vi "Test-Elevator-Commands.vi"() -> ()   [LabVIEW 2014, in "Comp Elevator.lvlib"]
uses:
  Comp Elevator.lvlib
  Robot/Elevator/Elevator Command/EL-Go to Height/EL-Go To Height Class/Parameters.ctl
  Robot/Elevator/Elevator Class/Elevator State.ctl
  Robot/Elevator/Elevator State Receiver Class/Elevator State Receiver.lvclass
  <vilib>/Rock Robotics/WPI/DriverStation/WPI_DriverStationRobotMode2.ctl
  Robot/Elevator/Elevator State Receiver Messages/Update Elevator State Msg/Update Elevator State Msg.lvclass
  Robot/Elevator/Elevator Messages/Request Current State Msg/Request Current State Msg.lvclass
  Robot/Elevator/Elevator Command/EL-Go to Height/EL-Go To Height Class/EL-Go To Height.lvclass
  Robot Actor Framework/System Actor/System Actor Messages/Start Command Msg/Start Command Msg.lvclass/Start Command Msg.ctl
  <vilib>/ActorFramework/Message Enqueuer/Message Enqueuer.lvclass/Message Enqueuer.ctl
  Robot/Elevator/Elevator Messages/Set Rate (Percent) Msg/Set Rate (Percent) Msg.lvclass/Set Rate (Percent) Msg.ctl
  <vilib>/ActorFramework/Message Enqueuer/Enqueue.vi
  Dev Robot/Robot Global Data.vi
  <vilib>/ActorFramework/Message Priority Queue/Priority Enqueue.vi
  Robot Actor Framework/System Actor/System Actor Messages/Update Tuning from File Msg/Update Tuning from File Msg.lvclass
  Robot Actor Framework/System Actor/System Actor Messages/Start Command Msg/Start Command Msg.lvclass
  Robot/Elevator/Elevator Messages/Set Rate (Percent) Msg/Set Rate (Percent) Msg.lvclass
  Robot Actor Framework/System Actor/System Actor Messages/Stop Command Msg/Stop Command Msg.lvclass
  <vilib>/ActorFramework/Stop Msg/Stop Msg.lvclass
  Robot Actor Framework/Command Actor/Command Actor Class/Command Actor.lvclass
  Robot Actor Framework/Utilities/Utilities.lvlib
  <vilib>/ActorFramework/Actor/Actor.lvclass
  Robot/Elevator/Elevator Class/Elevator.lvclass
panel:
  out "Delivery Notifier Error":errorcluster
  in  "Stop Command":bool=TRUE
  in  "Manual Elevate":enum32{"Up", "Hold", "Down"}(radio)=enum."Hold"
  out "error out":errorcluster
  out "Elevator State":T1 {"Current Elevation" scale=0.0..100.0; "Current Travel Rate" scale=-1.0..1.0}
  out "Start Command error out":errorcluster
  out "Command Running":bool
  in  "Fire Commamd":bool
  in  "Command Parameters":enum32{"No Command", "Go To Height", "Page 2"}(tab)
  in  "EL-GTH-Parameters":T2={"Target Height"=0.0, "Elevator State Loop (ms)"=20, "Up Rate (Percentage)"=1.0, "Down Rate (Percentage)"=-1.0}
  in  "Command":T3(radio)
  in  "Test Loop":u32=75
  out "Enable Tele":bool caption="Enabled Teleop"
  in  "Stop Test Loop 1":bool=TRUE
  in  "Finish Test":bool=TRUE
  in  "Start Test":bool=TRUE
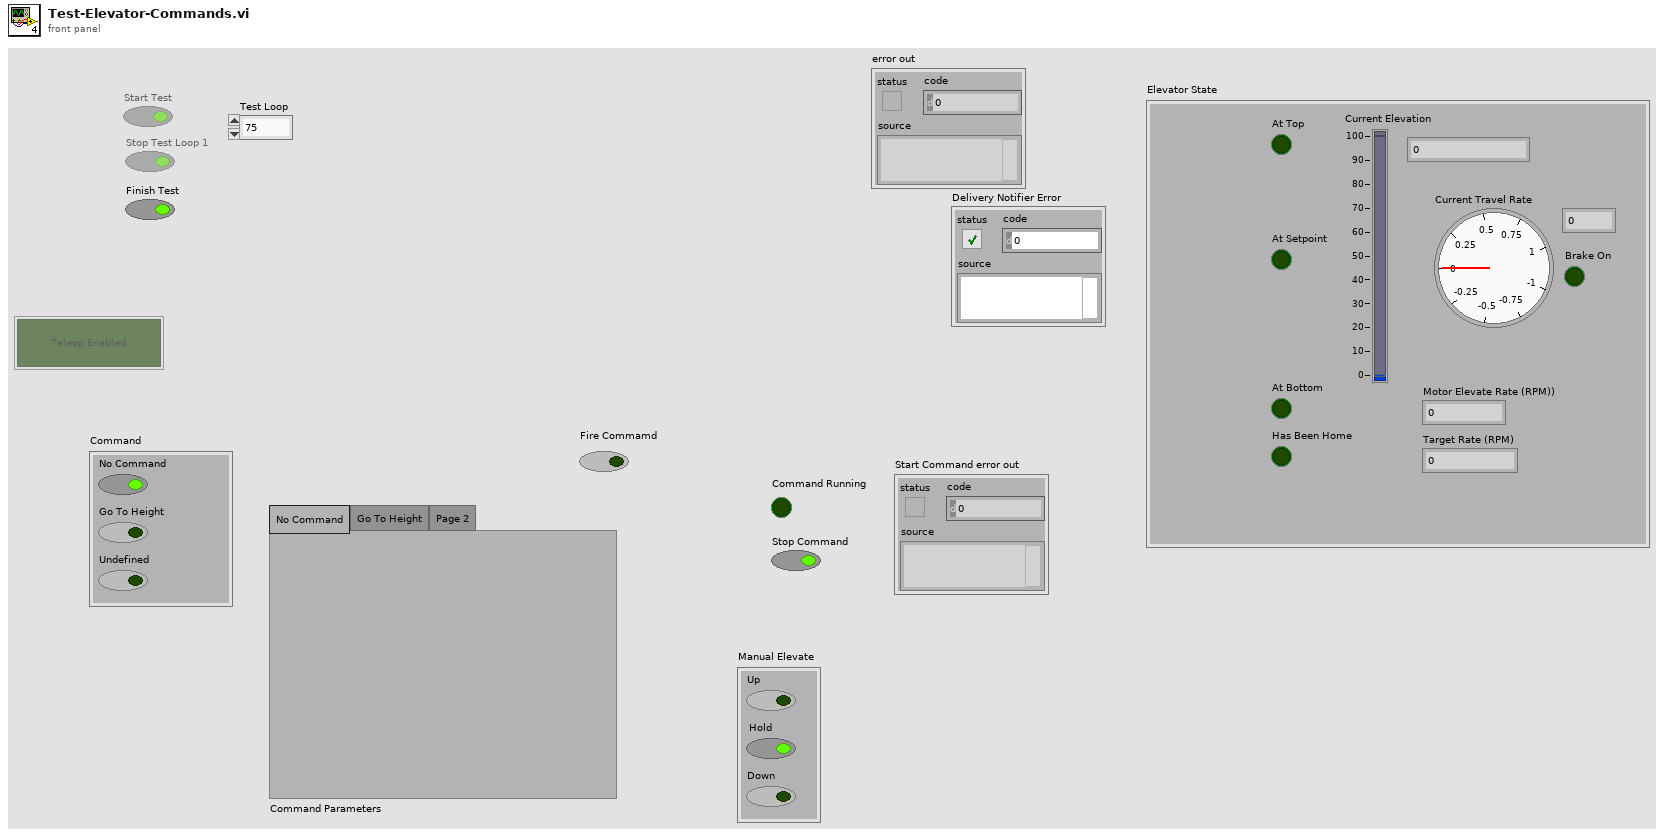
[diagram p1: front panel]
types:
  T1 = typedef "Elevator.lvlib/Elevator.lvclass/Elevator State.ctl" = cluster{"At Bottom":bool, "At Top":bool, "At Setpoint":bool, "Target Rate (RPM)":dbl, "Current Travel Rate":dbl, "Current Elevation":dbl, "Brake On":bool, "Motor Elevate Rate (RPM))":dbl, "Has Been Home":bool}
  T2 = typedef "Elevator.lvlib/EL-Go To Height.lvlib/EL-Go To Height.lvclass/Parameters.ctl" = cluster{"Target Height":dbl, "Elevator State Loop (ms)":u32, "Up Rate (Percentage)":dbl, "Down Rate (Percentage)":dbl}
  T3 = enum32{"No Command", "Go To Height", "Undefined"}
  T4 = enum8{"Enabled", "Disabled", "Disabled and Grayed Out"}
  T5 = typedef "WPI_DriverStationRobotMode2.ctl" = enum16{"Autonomous Disabled", "Autonomous Enabled", "Teleop Disabled", "Teleop Enabled", "Disconnected", "Finish", "Test Disabled", "Test Enabled", "Emergency Stopped"}
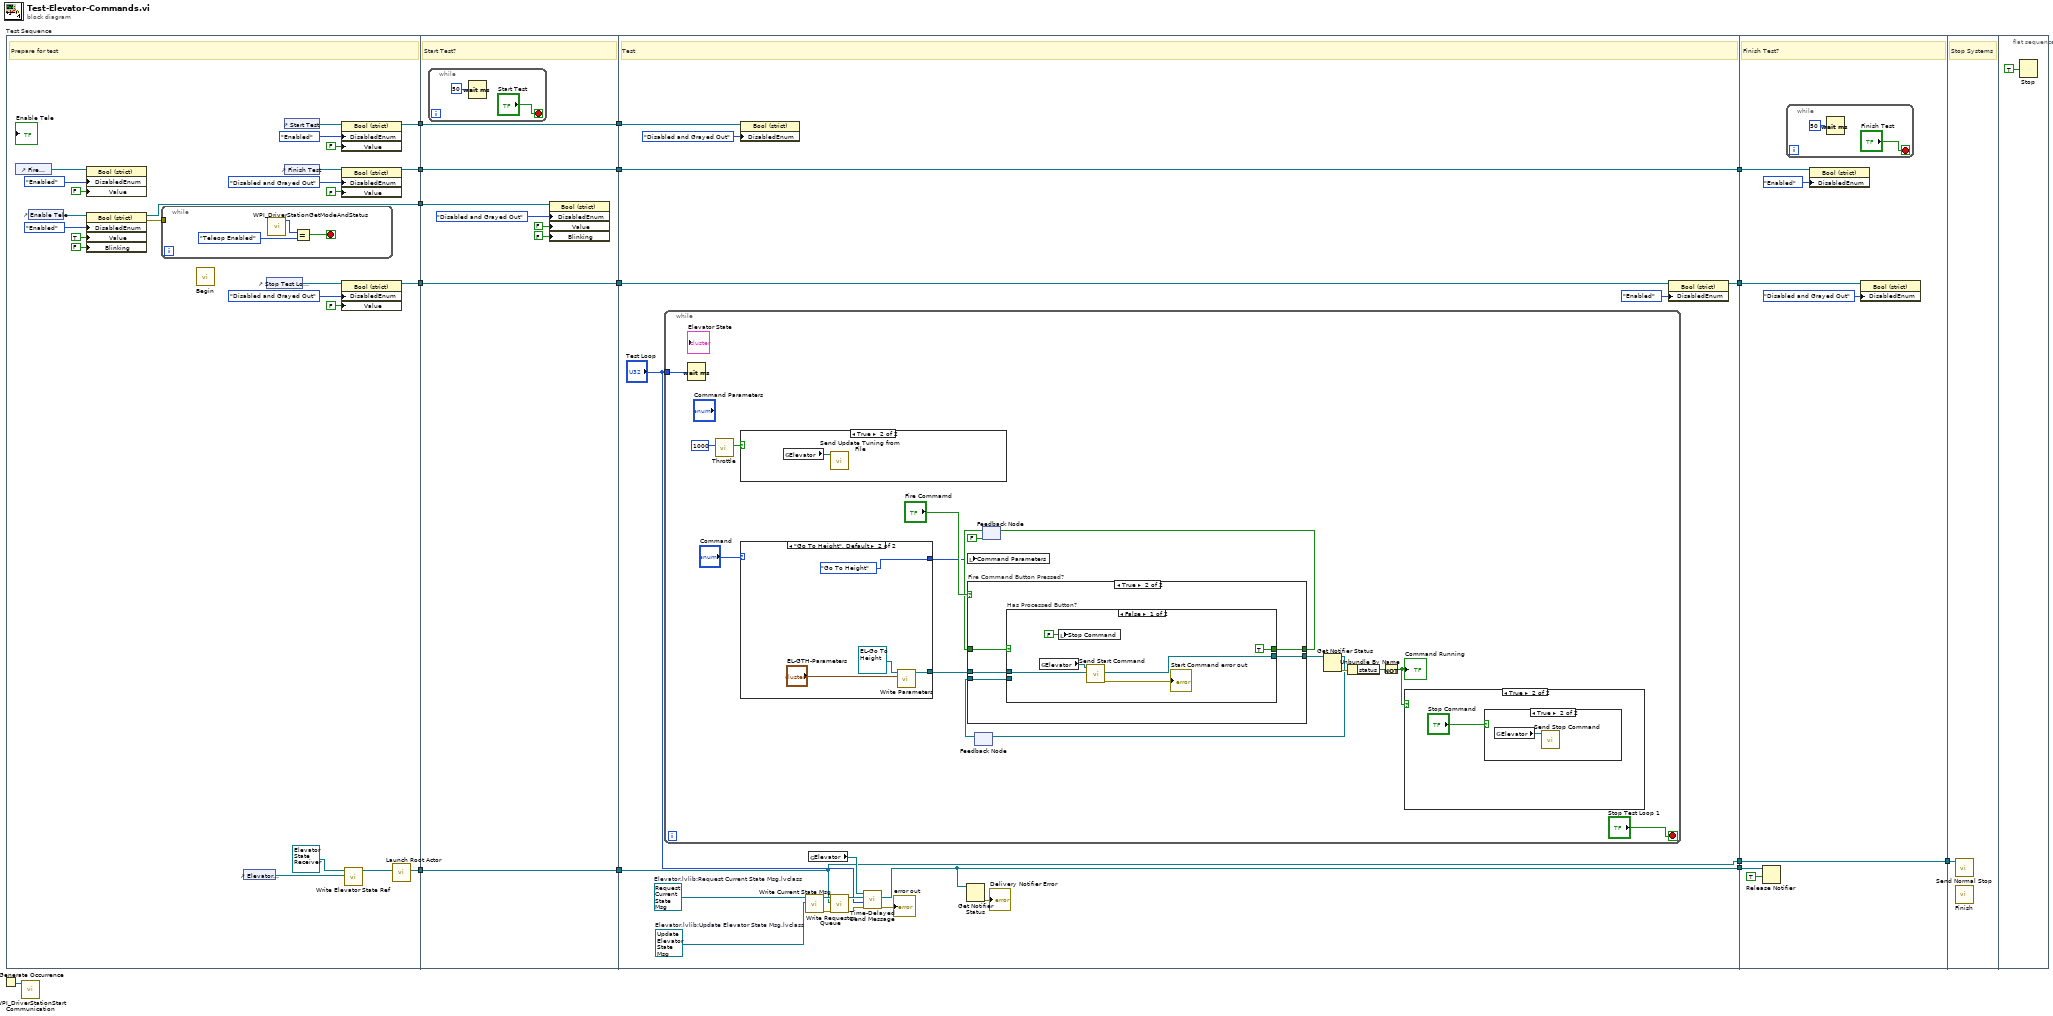
[diagram p0: block diagram]
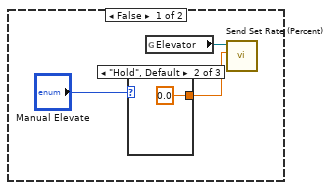
[diagram p2: hidden frame]
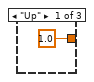
[diagram p3: hidden frame]
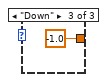
[diagram p4: hidden frame]
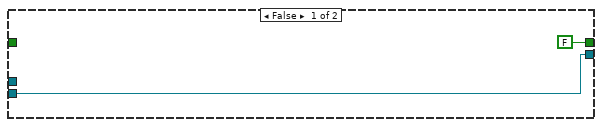
[diagram p7: hidden frame]
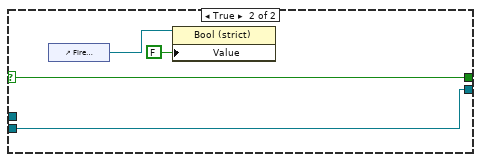
[diagram p8: hidden frame]
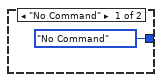
[diagram p9: hidden frame]
diagram:
  n1 = Generate Occurrence() -> (w15:refnum<k4>)
  n2 = flat-sequence "Test Sequence" {
    tunnel: [w31] -> w14
    tunnel: [w30] -> w12
    tunnel: [w29] -> w7
    tunnel: [w23] -> w6
    tunnel: [w19] -> w5
    tunnel: w14 -> [w51]
    tunnel: [w51] -> w13
    tunnel: w12 -> [w50]
    tunnel: [w50] -> w11
    tunnel: [w49] -> w8
    tunnel: w7 -> [w49]
    tunnel: w6 -> [w48]
    tunnel: w5 -> [w44]
    tunnel: [w44] -> w4
    tunnel: w13 -> [w71]
    tunnel: w11 -> [w69]
    tunnel: [w67] -> w10
    tunnel: [w66] -> w9
    tunnel: w8 -> [w66]
    tunnel: w4 -> [w59]
    tunnel: [w55] -> w3
    tunnel: [w59] -> w1
    tunnel: w10 -> [w126]
    tunnel: w9 -> [w123]
    tunnel: w3 -> [w122]
    tunnel: [w120] -> w2
    tunnel: w1 -> [w120]
    tunnel: w2 -> [w129]
    frame #0 {
      # "Prepare for test"
      n3 = control-ref of="Fire Commamd"() -> (w20:refnum<vi>)
      n4 = control-ref of="Enable Tele"() -> (w28:refnum<vi>)
      n5 = property class="Bool (strict)"(reference=w20, "DisabledEnum"=T4."Enabled" ("Disabled"), "Value"=FALSE) -> ()  [unwired: 1 in, 2 out]
      n6 = property class="Bool (strict)"(reference=w28, "DisabledEnum"=T4."Enabled" ("Disabled"), "Value"=TRUE, "Blinking"=FALSE) -> (reference out=w23:refnum<vi>, error out=w25:errorcluster)  [unwired: 1 in]
      n7 = while {
        tunnel: w25 -> [_]
        stop <- w41 stop-if-true
        n8 = call <vilib>:"WPI_DriverStationGetModeAndStatus.vi"() -> ("Robot Mode"=w43:T5)  [unwired: 10 in, 1 out]
        n9 = Equal?(x=w43, y=WPI_DriverStationRobotMode2."Teleop Enabled") -> (x = y?=w41:bool)
      }
      n10 = call "Begin.vi"() -> ()  [unwired: 11 in, 1 out]
      n11 = control-ref of="Elevator State"() -> (w16:refnum<vi>)
      n12 = control-ref of="Stop Test Loop 1"() -> (w35:refnum<vi>)
      n13 = control-ref of="Start Test"() -> (w40:refnum<vi>)
      n14 = control-ref of="Finish Test"() -> (w34:refnum<vi>)
      n15 = property class="Bool (strict)"(reference=w40, "DisabledEnum"=T4."Enabled" ("Disabled"), "Value"=FALSE) -> (reference out=w31:refnum<vi>)  [unwired: 1 in, 1 out]
      n16 = property class="Bool (strict)"(reference=w34, "DisabledEnum"=T4."Disabled and Grayed Out" ("Disabled"), "Value"=FALSE) -> (reference out=w29:refnum<vi>)  [unwired: 1 in, 1 out]
      n17 = property class="Bool (strict)"(reference=w35, "DisabledEnum"=T4."Disabled and Grayed Out" ("Disabled"), "Value"=FALSE) -> (reference out=w30:refnum<vi>)  [unwired: 1 in, 1 out]
      n18 = call-dynamic "Write Elevator State Ref.vi"("Elevator State Ref"=w16, "Elevator State Receiver in"=refnum<class "Elevator State Receiver.lvclass"> refnum ("Elevator.lvlib:Elevator State Receiver.lvclass")) -> ("Elevator State Receiver out"=w17:refnum<class "Elevator State Receiver.lvclass">)  [unwired: 8 in, 1 out]
      n19 = call <vilib>:"Launch Root Actor.vi"("Actor"=w17) -> ("Actor's Enqueuer"=w19:refnum<class "Message Enqueuer.lvclass">)  [unwired: 9 in, 1 out]
    }
    frame #1 {
      # "Start Test?"
      n20 = while {
        stop <- "Start Test" stop-if-true
        n21 = Wait (ms)(milliseconds to wait=u32 50) -> ()  [unwired: 1 out]
      }
      n22 = property class="Bool (strict)"(reference=w48, "DisabledEnum"=T4."Disabled and Grayed Out" ("Disabled"), "Value"=FALSE, "Blinking"=FALSE) -> ()  [unwired: 1 in, 2 out]
    }
    frame #2 {
      w65 = refnum<class "Request Current State Msg.lvclass"> refnum  # Elevator.lvlib:Request Current State Msg.lvclass
      w63 = refnum<class "Update Elevator State Msg.lvclass"> refnum  # Elevator.lvlib:Update Elevator State Msg.lvclass
      # "Test"
      n23 = while {
        tunnel: "Test Loop" -> [w75]
        stop <- "Stop Test Loop 1" stop-if-true
        n24 = Wait (ms)(milliseconds to wait=w75) -> ()  [unwired: 1 out]
        n25 = call "Throttle.vi"("Throttle (ms)"=u32 1000) -> ("Past Throttle"=w76:bool)  [unwired: 10 in]
        n26 = case shown="True" w76 {
          frame False {
          }
          frame True {
            n27 = global read "Robot Global Data.vi" "Elevator"() -> (w97:refnum<class "Message Enqueuer.lvclass">)
            n28 = call "Send Update Tuning from File.vi"("Message Enqueuer"=w97) -> ()  [unwired: 9 in, 2 out]
          }
        }
        n29 = case shown="\"Go To Height\", Default" "Command" {
          tunnel: [_ w117] -> w83
          tunnel: [enum32{"No Command", "Go To Height", "Page 2"}."No Command" ("Command Parameters") enum32{"No Command", "Go To Height", "Page 2"}."Go To Height" ("Command Parameters")] -> w73
          frame "No Command" {
          }
          frame "Go To Height", Default {
            n30 = call-dynamic "Write Parameters.vi"("Parameters"="EL-GTH-Parameters", "EL-Go To Height in"=refnum<class "EL-Go To Height.lvclass"> refnum ("Elevator.lvlib:EL-Go To Height.lvlib:EL-Go To Height.lvclass")) -> ("EL-Go To Height out"=w117:refnum<class "EL-Go To Height.lvclass">)  [unwired: 8 in, 1 out]
          }
        }
        n31 = local write "Command Parameters"(w73) -> ()
        n32 = feedback #1() -> (w78:refnum<notifier>)  [unwired: 1 in]
        n33 = feedback #2(FALSE) -> (w84:bool)
        n34 = case "Fire Command Button Pressed?" shown="True" "Fire Commamd" {
          tunnel: w84 -> [_ w104]
          tunnel: w83 -> [_ w103]
          tunnel: [FALSE w102] -> w82
          tunnel: [w98 w101] -> w79
          tunnel: w78 -> [w98 w100]
          frame False {
          }
          frame True {
            n35 = case "Has Processed Button?" shown="False" w104 {
              selector: w104 -> [_ w114]
              tunnel: w103 -> [w109 _]
              tunnel: [TRUE w114] -> w102
              tunnel: [w106 w113] -> w101
              tunnel: w100 -> [_ w113]
              frame False {
                n36 = global read "Robot Global Data.vi" "Elevator"() -> (w110:refnum<class "Message Enqueuer.lvclass">)
                n37 = local write "Stop Command"(FALSE ("Stop Command")) -> ()
                n38 = call "Send Start Command.vi"("Robot Actors.lvlib:Command.lvlib:Command.lvclass"=w109, "Message Enqueuer"=w110) -> ("error out"=→"Start Command error out":errorcluster, "Command notifier"=w106:refnum<notifier>)  [unwired: 7 in, 1 out]
              }
              frame True {
                n39 = control-ref of="Fire Commamd"() -> (w112:refnum<vi>)
                n40 = property class="Bool (strict)"(reference=w112, "Value"=FALSE) -> ()  [unwired: 1 in, 2 out]
              }
            }
          }
        }
        n41 = feedback-in #2(w82) -> ()
        n42 = Get Notifier Status(notifier=w79) -> (notifier out=w72:refnum<notifier>, error out=w81:errorcluster)  [unwired: 1 in, 3 out]
        n43 = feedback-in #1(w72) -> ()
        n44 = Unbundle By Name(w81) -> ("status"=w80:bool)
        n45 = Not(x=w80) -> (.not. x?=w74:bool)
        "Command Running" <- w74
        n46 = case shown="True" w74 {
          frame False {
            n47 = case shown="\"Hold\", Default" "Manual Elevate" {
              tunnel: [1.0 0.0 -1.0] -> w89
              frame "Up" {
              }
              frame "Hold", Default {
              }
              frame "Down" {
              }
            }
            n48 = global read "Robot Global Data.vi" "Elevator"() -> (w90:refnum<class "Message Enqueuer.lvclass">)
            n49 = call "Send Set Rate (Percent).vi"("Percent"=w89, "Message Enqueuer"=w90) -> ()  [unwired: 8 in, 2 out]
          }
          frame True {
            n50 = case shown="True" "Stop Command" {
              frame False {
              }
              frame True {
                n51 = global read "Robot Global Data.vi" "Elevator"() -> (w96:refnum<class "Message Enqueuer.lvclass">)
                n52 = call "Send Stop Command.vi"("Message Enqueuer"=w96) -> ()  [unwired: 9 in, 2 out]
              }
            }
          }
        }
      }
      n53 = property class="Bool (strict)"(reference=w71, "DisabledEnum"=T4."Disabled and Grayed Out" ("Disabled")) -> ()  [unwired: 1 in, 2 out]
      n54 = call-dynamic "Write Current State Msg.vi"("Elevator.lvlib:Current State Msg.lvclass"=w63, "Request Current State Msg in"=w65) -> ("error out"=w57:errorcluster, "Request Current State Msg out"=w64:refnum<class "Request Current State Msg.lvclass">)  [unwired: 8 in]
      n55 = global read "Robot Global Data.vi" "Elevator"() -> (w61:refnum<class "Message Enqueuer.lvclass">)
      n56 = call-dynamic "Write Requestor Queue.vi"("error in (no error)"=w57, "Actor Framework:Message Enqueuer"=w59, "Request Current State Msg in"=w64) -> ("error out"=w56:errorcluster, "Request Current State Msg out"=w62:refnum<class "Request Current State Msg.lvclass">)  [unwired: 7 in]
      n57 = call <vilib>:"Time-Delayed Send Message.vi"("error in (no error)"=w56, "Milliseconds To Wait"="Test Loop", "Message"=w62, "Message Enqueuer"=w61) -> ("error out"=→"error out":errorcluster, "Delivery Notifier"=w55:refnum<notifier>)  [unwired: 6 in]
      n58 = Get Notifier Status(notifier=w55) -> (error out=→"Delivery Notifier Error":errorcluster)  [unwired: 1 in, 4 out]
      n59 = property class="Bool (strict)"(reference=w69, "DisabledEnum"=T4."Enabled" ("Disabled")) -> (reference out=w67:refnum<vi>)  [unwired: 1 in, 1 out]
    }
    frame #3 {
      # "Finish Test?"
      n60 = Release Notifier(notifier=w122, force destroy? (F)=TRUE) -> ()  [unwired: 1 in, 3 out]
      n61 = while {
        stop <- "Finish Test" stop-if-true
        n62 = Wait (ms)(milliseconds to wait=u32 50) -> ()  [unwired: 1 out]
      }
      n63 = property class="Bool (strict)"(reference=w123, "DisabledEnum"=T4."Enabled" ("Disabled")) -> ()  [unwired: 1 in, 2 out]
      n64 = property class="Bool (strict)"(reference=w126, "DisabledEnum"=T4."Disabled and Grayed Out" ("Disabled")) -> ()  [unwired: 1 in, 2 out]
    }
    frame #4 {
      # "Stop Systems"
      n65 = call <vilib>:"Send Normal Stop.vi"("Message Enqueuer"=w129) -> ()  [unwired: 10 in, 1 out]
      n66 = call "Finish.vi"() -> ()  [unwired: 8 in]
    }
    frame #5 {
      n67 = Stop(stop? (T)=TRUE) -> ()
    }
  }
  n68 = call <vilib>:"WPI_DriverStationStart Communication.vi"("occurrence"=w15) -> ()  [unwired: 1 in, 10 out]
